vi "Matlab.vi"(0 "ColorchocWin":u32(colorbox), 1 "error in":errorcluster, 3 "Boolean":bool, 4 "Ball Coordinates":cluster{"Array":dbl[], "Array 2":dbl[]}[](array[cluster]), 5 "LineStyle":u16, 6 "ColorchocLoose":u32(colorbox), 7 "MarkerStyle":u16, 8 "Path":path) -> (11 "Script":string, 12 "error out":errorcluster)   [LabVIEW 2025]
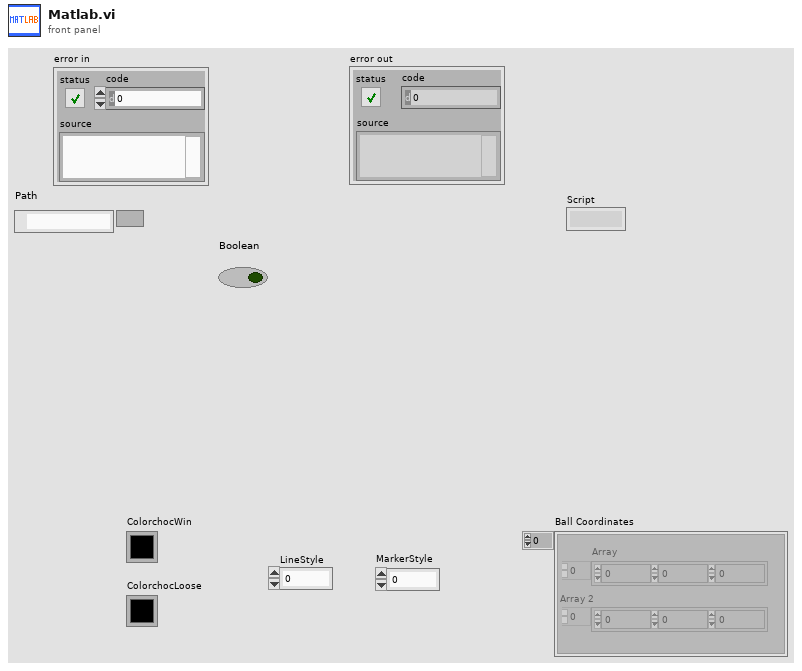
[diagram p1: front panel]
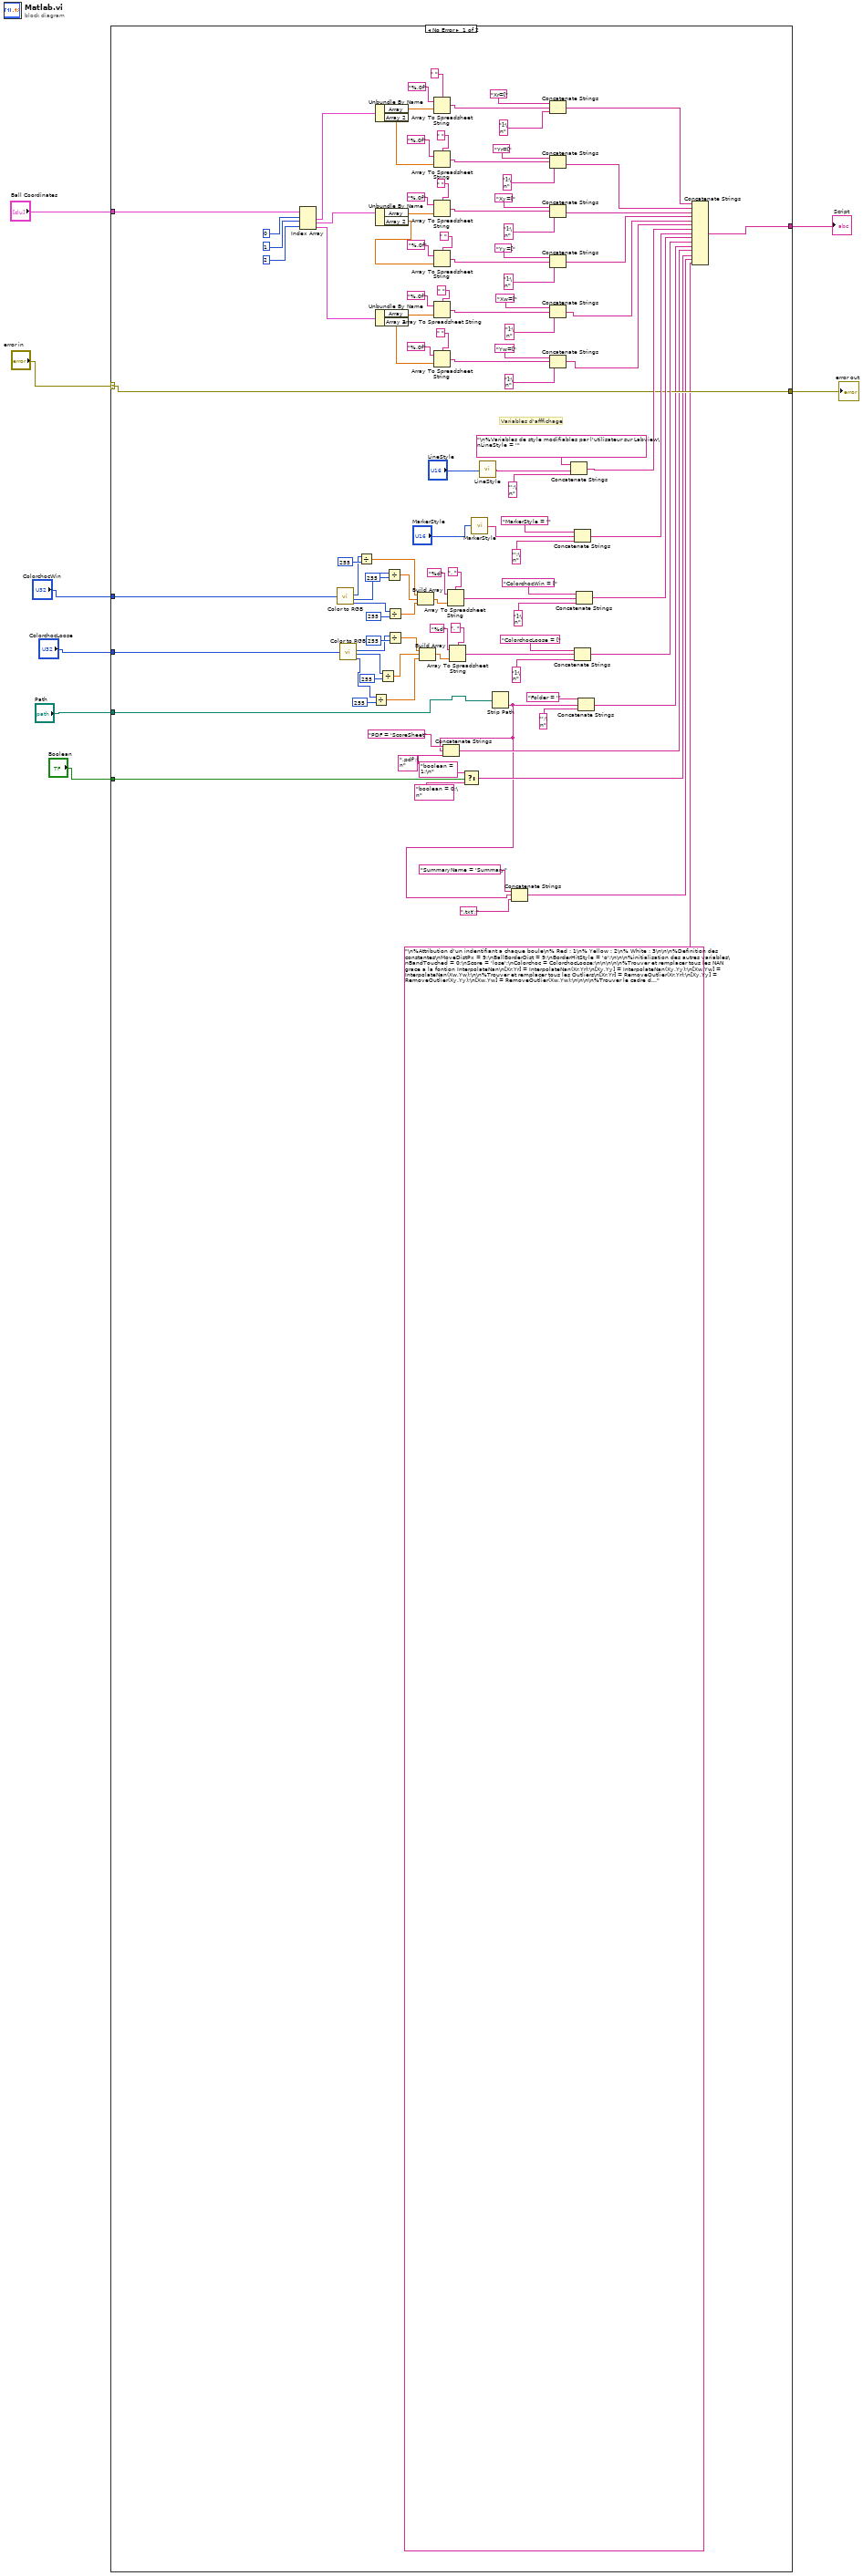
[diagram p0: block diagram]
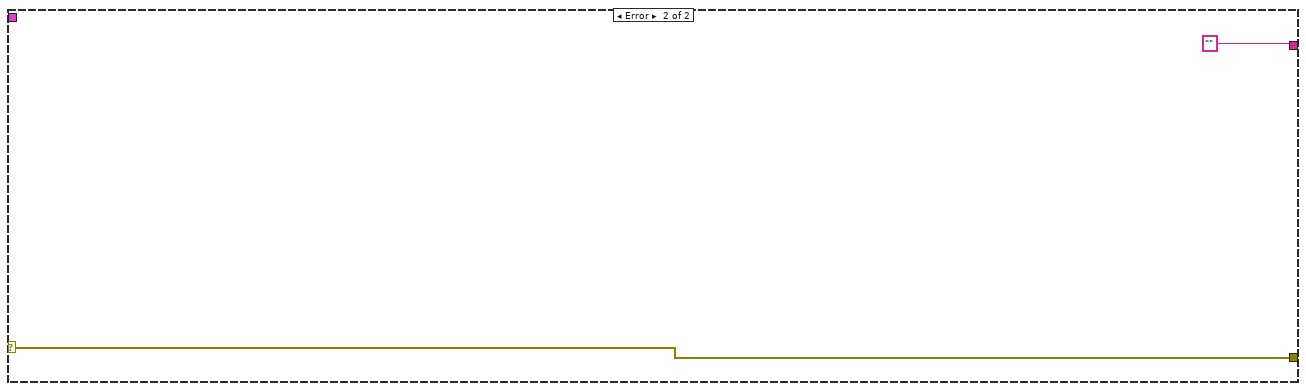
[diagram p2: hidden frame]
diagram:
  n1 = case shown="No Error" "error in" {
    selector: "error in" -> [w46 w120]
    tunnel: [w50 ""] -> w8
    tunnel: "Ball Coordinates" -> [w49 _]
    tunnel: "ColorchocWin" -> [w48 _]
    tunnel: "ColorchocLoose" -> [w47 _]
    tunnel: [w46 w120] -> w4
    tunnel: "Boolean" -> [w41 _]
    tunnel: "Path" -> [w9 _]
    frame No Error {
      # "Variables d'afffichage"
      n2 = Index Array(array=w49, index #1=0, index #2=1, index #3=2) -> (element #1=w78:cluster{"Array":dbl[], "Array 2":dbl[]}, element #2=w35:cluster{"Array":dbl[], "Array 2":dbl[]}, element #3=w33:cluster{"Array":dbl[], "Array 2":dbl[]})
      n3 = call <vilib>:"Color to RGB.vi"("Color"=w48) -> ("R"=w20:u8, "G"=w19:u8, "B"=w17:u8)  [unwired: 1 out]
      n4 = call <vilib>:"Color to RGB.vi"("Color"=w47) -> ("R"=w15:u8, "G"=w13:u8, "B"=w11:u8)  [unwired: 1 out]
      n5 = Divide(x=w20, y=255) -> (x/y=w21:dbl)
      n6 = Divide(x=w11, y=255) -> (x/y=w10:dbl)
      n7 = Unbundle By Name(w78) -> ("Array"=w77:dbl[], "Array 2"=w37:dbl[])
      n8 = Unbundle By Name(w35) -> ("Array"=w80:dbl[], "Array 2"=w36:dbl[])
      n9 = Unbundle By Name(w33) -> ("Array"=w79:dbl[], "Array 2"=w34:dbl[])
      n10 = Divide(x=w13, y=255) -> (x/y=w12:dbl)
      n11 = Divide(x=w19, y=255) -> (x/y=w18:dbl)
      n12 = Divide(x=w17, y=255) -> (x/y=w16:dbl)
      n13 = Divide(x=w15, y=255) -> (x/y=w14:dbl)
      n14 = Build Array(w21, w18, w16) -> (w58:dbl[])
      n15 = Build Array(w14, w12, w10) -> (w54:dbl[])
      n16 = Array To Spreadsheet String(delimiter (Tab)=" ", array=w77, 3:"%.0f") -> (spreadsheet string=w69:string)
      n17 = Array To Spreadsheet String(delimiter (Tab)=" ", array=w37, 3:"%.0f") -> (spreadsheet string=w63:string)
      n18 = Array To Spreadsheet String(delimiter (Tab)=" ", array=w80, 3:"%.0f") -> (spreadsheet string=w62:string)
      n19 = Array To Spreadsheet String(delimiter (Tab)=" ", array=w36, 3:"%.0f") -> (spreadsheet string=w61:string)
      n20 = Array To Spreadsheet String(delimiter (Tab)=" ", array=w79, 3:"%.0f") -> (spreadsheet string=w60:string)
      n21 = Array To Spreadsheet String(delimiter (Tab)=" ", array=w34, 3:"%.0f") -> (spreadsheet string=w59:string)
      n22 = Array To Spreadsheet String(delimiter (Tab)=", ", array=w58, 3:"%d") -> (spreadsheet string=w55:string)
      n23 = Array To Spreadsheet String(delimiter (Tab)=", ", array=w54, 3:"%d") -> (spreadsheet string=w51:string)
      n24 = Select(t="boolean = 1;\n", s=w41, f="boolean = 0;\n") -> (s? t:f=w38:string)
      n25 = call "MarkerStyle.vi"("Enum MarkerStyle"="MarkerStyle") -> ("MarkerStyle"=w83:string)
      n26 = call "LineStyle.vi"("Enum LineStyle"="LineStyle") -> ("LineStyle"=w81:string)
      n27 = Strip Path(path=w9) -> (name=w30:string)  [unwired: 1 out]
      n28 = Concatenate Strings("PDF = 'ScoreSheet", w30, ".pdf';\n") -> (w42:string)
      n29 = Concatenate Strings("SummaryName = 'Summary", w30, ".txt';") -> (w28:string)
      n30 = Concatenate Strings("Xr=[", w69, "];\n") -> (w97:string)
      n31 = Concatenate Strings("Yr=[", w63, "];\n") -> (w96:string)
      n32 = Concatenate Strings("Xy=[", w62, "];\n") -> (w95:string)
      n33 = Concatenate Strings("Yy=[", w61, "];\n") -> (w94:string)
      n34 = Concatenate Strings("Xw=[", w60, "];\n") -> (w93:string)
      n35 = Concatenate Strings("Yw=[", w59, "];\n") -> (w92:string)
      n36 = Concatenate Strings("\n%Variables de style modifiables par l'utilisateur sur Labview\nLineStyle = '", w81, "';\n") -> (w91:string)
      n37 = Concatenate Strings("MarkerStyle = '", w83, "';\n") -> (w90:string)
      n38 = Concatenate Strings("ColorchocLoose = [", w51, "];\n") -> (w88:string)
      n39 = Concatenate Strings("ColorchocWin = [", w55, "];\n") -> (w89:string)
      n40 = Concatenate Strings("Folder = '", w30, "';\n") -> (w45:string)
      n41 = Concatenate Strings(w97, w96, w95, w94, w93, w92, w91, w90, w89, w88, w45, w42, w38, w28, "\n%Attribution d'un indentifiant a chaque boule\n% Red : 1\n% Yellow : 2\n% White : 3\n\n\n%Definition des constantes\nMoveDistPx = 9;\nBallBorderDist = 9;\nBorderHitStyle = 'o';\n\n\n%initialisation des autres variables\nBandTouched = 0;\nScore = 'lose';\nColorchoc = ColorchocLoose;\n\n\n\n\n%Trouver et remplacer tous les NAN grace a la fontion InterpolateNan\n[Xr,Yr] = InterpolateNan(Xr,Yr);\n[Xy,Yy] = InterpolateNan(Xy,Yy);\n[Xw,Yw] = InterpolateNan(Xw,Yw);\n\n%Trouver et remplacer tous les Outliers\n[Xr,Yr] = RemoveOutlier(Xr,Yr);\n[Xy,Yy] = RemoveOutlier(Xy,Yy);\n[Xw,Yw] = RemoveOutlier(Xw,Yw);\n\n\n\n%Trouver le cadre du billard\n[Xmin, Xmax, Ymin,Ymax] = GetFrame(Xr,Yr,Xy,Yy,Xw,Yw);\n\n%Hauteur de notre billard\nH = Ymax-Ymin;\n\n\nX_frame = [Xmin Xmax Xmax Xmin Xmin];\nY_frame = [Ymin Ymin Ymax Ymax Ymin];\n\n\n%Donne le nombre et l'ordre des balles qui ont bouge\n[FirstBall, SecondBall, LastBall, NbBallsMoved] = GetBallMoveOrder(Xr, Yr, Xy, Yy, Xw, Yw, MoveDistPx);\n\n%Nous donne l'indice a laquelle chaque boule commence a bouger\n[FirstMoveIdxR, MoveDistR] = GetFirstMoveIdx(Xr,Yr, MoveDistPx);\n[FirstMoveIdxY, MoveDistY] = GetFirstMoveIdx(Xy,Yy, MoveDistPx);\n[FirstMoveIdxW, MoveDistW] = GetFirstMoveIdx(Xw,Yw, MoveDistPx);\nOrderIdx = sort([FirstMoveIdxR, FirstMoveIdxY, FirstMoveIdxW]);\n\n\n\n\n%Distance totale parcourue par chaque balle\nPathLengthR = GetBallPathLength(Xr,Yr);\nPathLengthY = GetBallPathLength(Xy,Yy);\nPathLengthW = GetBallPathLength(Xw,Yw);\n\n\n\n\n\n%Partie visuelle\nfigure\n\nhold on\n\naxis off\n\n%Tracer la trajectoire de chaque boule en n'oubliant pas d'inverser les coordonees Y\nplot(Xr, H-Yr, 'r', 'LineStyle', LineStyle, 'Marker', MarkerStyle);\nplot(Xy, H-Yy, 'Color', [0.9 0.7 0],'LineStyle', LineStyle, 'Marker', MarkerStyle); %couleur : jaune fonce \nplot(Xw, H-Yw, 'b','LineStyle', LineStyle, 'Marker', MarkerStyle);\nplot(X_frame, H-Y_frame, 'k');\n\n%Illustration des positions initiales des boules\nplot(Xr(1), H-Yr(1), 'Marker', 'h', 'MarkerSize', 15, 'MarkerEdgeColor', 'r');\nplot(Xy(1), H-Yy(1), 'Marker', 'h', 'MarkerSize', 15, 'MarkerEdgeColor', [0.9 0.7 0]);\nplot(Xw(1), H-Yw(1), 'Marker', 'h', 'MarkerSize', 15, 'MarkerEdgeColor', 'b');\n\n\n%Dans le cas ou la balle rouge est tappee en premier\nif FirstBall == 1\n\n    [IdxTouchR, offset] = GetTouchIdx(Xr,Yr,Xmin, Xmax, Ymin, Ymax, BallBorderDist);\n\n    %Masque servant a isoler les rebonds valides\n    MaskBetween = IdxTouchR > OrderIdx(2) & IdxTouchR < OrderIdx(3);\n    IdxTouchR_between = IdxTouchR(MaskBetween);    \n\n    %Renvoie le nombre de bord qui sont touches par la boule principale apres avoir tape la premiere boule\n    %et avant d'avoir tappe la 2eme\n    ValidBoarderTouch = length(IdxTouchR_between);\n\n     %Conditions necessaires pour gagner\n    if NbBallsMoved == 3 && ValidBoarderTouch >= 3\n        Score = 'Win';\n        Colorchoc = ColorchocWin;\n    end\n\n    %Trace les contacts entre les bords et la boule\n    %plot(Xr(IdxTouchR + offset), H-Yr(IdxTouchR + offset), 'Marker', BorderHitStyle, 'MarkerSize', 15, 'MarkerEdgeColor', Colorchoc, 'LineStyle', 'none');\n    plot(Xr(IdxTouchR_between + offset), H - Yr(IdxTouchR_between + offset), 'Marker', BorderHitStyle, 'MarkerSize', 15, 'MarkerEdgeColor', Colorchoc, 'LineStyle', 'none');\n\n\n    %Ecriture sur d'une partie des resultats\n    text(Xmin, (H-Ymax)-0.05*H,'Score sheet for \"red\"');\n    text(Xmin + (Xmax - Xmin)*0.8, (H-Ymax)-0.07*H,{[num2str(NbBallsMoved) ' ball(s) touched'],[num2str(ValidBoarderTouch) ' band(s) touched']})\n\n\n   \nend\n\n%Idem si c'est la boule jaune qui est tappee en premier\nif FirstBall == 2\n\n    [IdxTouchY, offset] = GetTouchIdx(Xy,Yy,Xmin, Xmax, Ymin, Ymax, BallBorderDist);\n\n    MaskBetween = IdxTouchY > OrderIdx(2) & IdxTouchY < OrderIdx(3);\n    IdxTouchY_between = IdxTouchY(MaskBetween);\n   \n    ValidBoarderTouch = length(IdxTouchY_between);\n\n    if NbBallsMoved == 3 && ValidBoarderTouch >= 3\n        Score = 'Win';\n        Colorchoc = ColorchocWin;\n    end\n\n    plot(Xy(IdxTouchY_between + offset), H - Yy(IdxTouchY_between + offset), 'Marker', BorderHitStyle, 'MarkerSize', 15, 'MarkerEdgeColor', Colorchoc, 'LineStyle', 'none');\n\n    text(Xmin, (H-Ymax)-0.05*H,'Score sheet for \"yellow\"');\n    text(Xmin + (Xmax - Xmin)*0.8,(H-Ymax)-0.07*H,{[num2str(NbBallsMoved) ' ball(s) touched'],[num2str(ValidBoarderTouch) ' band(s) touched']})\n\n\nend\n\n\n\n%Idem si c'est la boule blanche qui est tappee en premier\nif FirstBall == 3\n\n    [IdxTouchW, offset] = GetTouchIdx(Xw,Yw,Xmin, Xmax, Ymin, Ymax, BallBorderDist);\n\n    MaskBetween = IdxTouchW > OrderIdx(2) & IdxTouchW < OrderIdx(3);\n    IdxTouchW_between = IdxTouchW(MaskBetween);\n   \n    ValidBoarderTouch = length(IdxTouchW_between);\n\n    if NbBallsMoved == 3 && ValidBoarderTouch >= 3\n        Score = 'Win';\n        Colorchoc = ColorchocWin;\n    end\n\n    plot(Xw(IdxTouchW_between + offset), H - Yw(IdxTouchW_between + offset), 'Marker', BorderHitStyle, 'MarkerSize', 15, 'MarkerEdgeColor', Colorchoc, 'LineStyle', 'none');\n   \n    text(Xmin, (H-Ymax)-0.05*H,'Score sheet for \"white\"');\n    text(Xmin + (Xmax - Xmin)*0.8,(H-Ymax)-0.07*H,{[num2str(NbBallsMoved) ' ball(s) touched'],[num2str(ValidBoarderTouch) ' band(s) touched']})\n\n\nend\n\n\n%Ecriture du titre et du reste des resultats de la partie\ntitle(['Scores sheet - ' Folder ' - (' char(datetime('now')) ')'], 'FontSize', 15)\n\n%Utilisation de num2str pour convertir en string et int32 pour convertir en\n%int\ntext(Xmin + (Xmax - Xmin)*0.2, (H-Ymax)-0.2*H,['red_d:' num2str(int32(PathLengthR)) 'px']);\ntext(Xmin + (Xmax - Xmin)*0.45, (H-Ymax)-0.2*H,['yellow_d:' num2str(int32(PathLengthY)) 'px']);\ntext(Xmin + (Xmax - Xmin)*0.7,(H-Ymax)-0.2*H,['white_d:' num2str(int32(PathLengthW)) 'px']);\n\n\n\n%Ecriture du score\ntext(Xmin, (H-Ymax)-0.1*H, ['---' Score '---']);\n\nhold off\n\n\n%Ecriture dans le PDF\n\n%F(irstball)\nif FirstBall == 1\n    f_char = 'r';\nelseif FirstBall == 2\n    f_char = 'y';\nelseif FirstBall == 3\n    f_char = 'w';\nelse\n    f_char = '?';\nend\n\n\n%S(core)\nif strcmpi(Score,'Win')\n    s_char = 'w';\nelse\n    s_char = 'l';\nend\n\n\n%Sauvegarde du PDF ScoreSheetXX.pdf\nfilenamePDF = sprintf('ScoreSheet%s.pdf', Folder);\nsaveas(gcf, filenamePDF);\n\n\nif boolean\nopen(PDF);\nend\n\n\n%Chaine finale\nMessage = sprintf(\"f:%s; s:%s; n:%d; b:%d; rb:%d; yb:%d; wb:%d;\", f_char, s_char, NbBallsMoved, ValidBoarderTouch, int32(PathLengthR), int32(PathLengthY), int32(PathLengthW));\n\n\n%Sauvegarde du SummaryXX.txt\nfilenameTXT = sprintf(SummaryName, Folder);\nfid = fopen(filenameTXT, 'w');\nfprintf(fid, \"%s\\n\", Message);\nfclose(fid);\n") -> (w50:string)
    }
    frame Error {
    }
  }
  "Script" <- w8
  "error out" <- w4
